vi "ODE_quaternion.vi"() -> ()   [LabVIEW 2018]
uses:
  <vilib>/robotics/Kinematics/Quaternion.ctl
  <vilib>/Analysis/_algsub.llb/Vector Norm.vi
  <vilib>/Analysis/_algsub.llb/Real Vector Norm.vi
  <vilib>/Analysis/baseanly.llb/Outer Product.vi
  <vilib>/Analysis/baseanly.llb/Real Outer Product.vi
  <vilib>/robotics/Kinematics/Create Lie Group Matrix.vi
  <vilib>/imath/engines/lvmath2/RunTimeEngine/Managers/WorkSpace/UID Generator.vi
  <vilib>/imath/engines/lvmath2/RunTimeEngine/IndexRead/NIMS V(S).vi
  <instcachedir>/0/NIMS V(S)_0488751826AF41519A22953C041130DC.lvgen/NIMS V(S)_0488751826AF41519A22953C041130DC_002.vi
  <vilib>/imathl/engines/lvmath/Functions/Error Handling/Create Error.vi
  <vilib>/imath/engines/lvmath2/RunTimeEngine/RunTimeType/NIMS_RunTimeType_From StrictType (excl LVString).vi
  <instcachedir>/0/NIMS_RunTimeType_From StrictType (excl LVString)_E7E34A65C99947108168652BAD14964D.lvgen/NIMS_RunTimeType_From StrictType (excl LVString)_E7E34A65C99947108168652BAD14964D_000.vi
  <vilib>/imath/engines/lvmath2/RunTimeEngine/LocalVariableDefStatement/MC_LocalVariableDefStatement_Display.vi
  <vilib>/imath/engines/lvmath2/RunTimeEngine/ArithmeticOperatorToken/NIMS_ArithmeticOperator_multmx(M,CV)-internal.vi
  <instcachedir>/0/NIMS_ArithmeticOperator_multmx(M,CV)-internal_5287250D8D1D4A3E9F77F5DF08D432E0.lvgen/NIMS_ArithmeticOperator_multmx(M,CV)-internal_5287250D8D1D4A3E9F77F5DF08D432E0_003.vi
  <instcachedir>/0/NIMS V(S)_0488751826AF41519A22953C041130DC.lvgen/NIMS V(S)_0488751826AF41519A22953C041130DC_000.vi
  <vilib>/imath/engines/lvmath2/RunTimeEngine/Managers/SymbolTable/Clear UID.vi
  <vilib>/imath/engines/lvmath2/RunTimeEngine/NodeEndStatement/NIMS_NodeEndStatement_Output.vi
  <instcachedir>/0/NIMS_NodeEndStatement_Output_53EC0D466D134D7ABD903AC30B43404B.lvgen/NIMS_NodeEndStatement_Output_53EC0D466D134D7ABD903AC30B43404B_005.vi
  <vilib>/imath/engines/lvmath2/RunTimeEngine/ErrorHandling/NIMS_Finalize Error.vi
  <vilib>/Analysis/Matrix/Numeric/Multiply/Multiply.vi
  <vilib>/Analysis/Matrix/Numeric/Multiply/Multiply - RM,R.vi
  <vilib>/Analysis/Matrix/Numeric/Multiply/Multiply - R,RM.vi
  <vilib>/Analysis/Matrix/Numeric/Add/Add.vi
  <vilib>/Analysis/Matrix/Numeric/Add/Add - RM,RM.vi
  <vilib>/Analysis/Matrix/Numeric/Conversions/Matrix To Array - RM.vi
  <vilib>/imath/engines/lvmath2/RunTimeEngine/IndexRead/NIMS M(S,S).vi
  <instcachedir>/0/NIMS M(S,S)_AC51E74150A542F7991B9634C66F3096.lvgen/NIMS M(S,S)_AC51E74150A542F7991B9634C66F3096_000.vi
  <vilib>/imath/engines/lvmath2/RunTimeEngine/BuiltInFunctions/abs/NIMS_abs(signed).vi
  <instcachedir>/0/NIMS_abs(signed)_C4FCB8E6058B49B797C7C8D53CA5F6EC.lvgen/NIMS_abs(signed)_C4FCB8E6058B49B797C7C8D53CA5F6EC_000.vi
  <vilib>/imath/engines/lvmath2/RunTimeEngine/BuiltInFunctions/atan2/NIMS_atan2.vi
  <instcachedir>/0/NIMS_atan2_A91AA4A7D42247EDBE8F76DB99AF04A4.lvgen/NIMS_atan2_A91AA4A7D42247EDBE8F76DB99AF04A4_002.vi
  <vilib>/imath/engines/lvmath2/RunTimeEngine/ErrorHandling/NIMS_Create Error From Enums.vi
  <vilib>/imath/engines/lvmath2/RunTimeEngine/BuiltInFunctions/cos/NIMS_cos(C).vi
  <instcachedir>/0/NIMS_cos(C)_96B8A70E6B8E4D29AD8526A89C8CF3DF.lvgen/NIMS_cos(C)_96B8A70E6B8E4D29AD8526A89C8CF3DF_001.vi
  <instcachedir>/0/NIMS_atan2_A91AA4A7D42247EDBE8F76DB99AF04A4.lvgen/NIMS_atan2_A91AA4A7D42247EDBE8F76DB99AF04A4_001.vi
  <vilib>/gmath/NI_Gmath.lvlib
  <vilib>/robotics/Kinematics/NI_Kinematics.lvlib
  <vilib>/imath/engines/lvmath2/RunTimeEngine/Managers/SymbolTable/NIMS_WorkSpace.lvlib
  <vilib>/Analysis/Matrix/NI_Matrix.lvlib
panel:
  out "E":dbl[](array[numeric])
  out "unit quaternion":T1
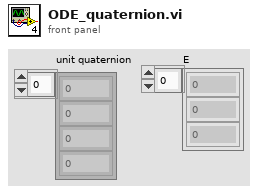
[diagram p1: front panel]
types:
  T1 = typedef "NI_Kinematics.lvlib/Quaternion.ctl" = dbl[]
  T2 = typedef "NI_Matrix.lvlib/RealMatrix.ctl" = dbl[][]
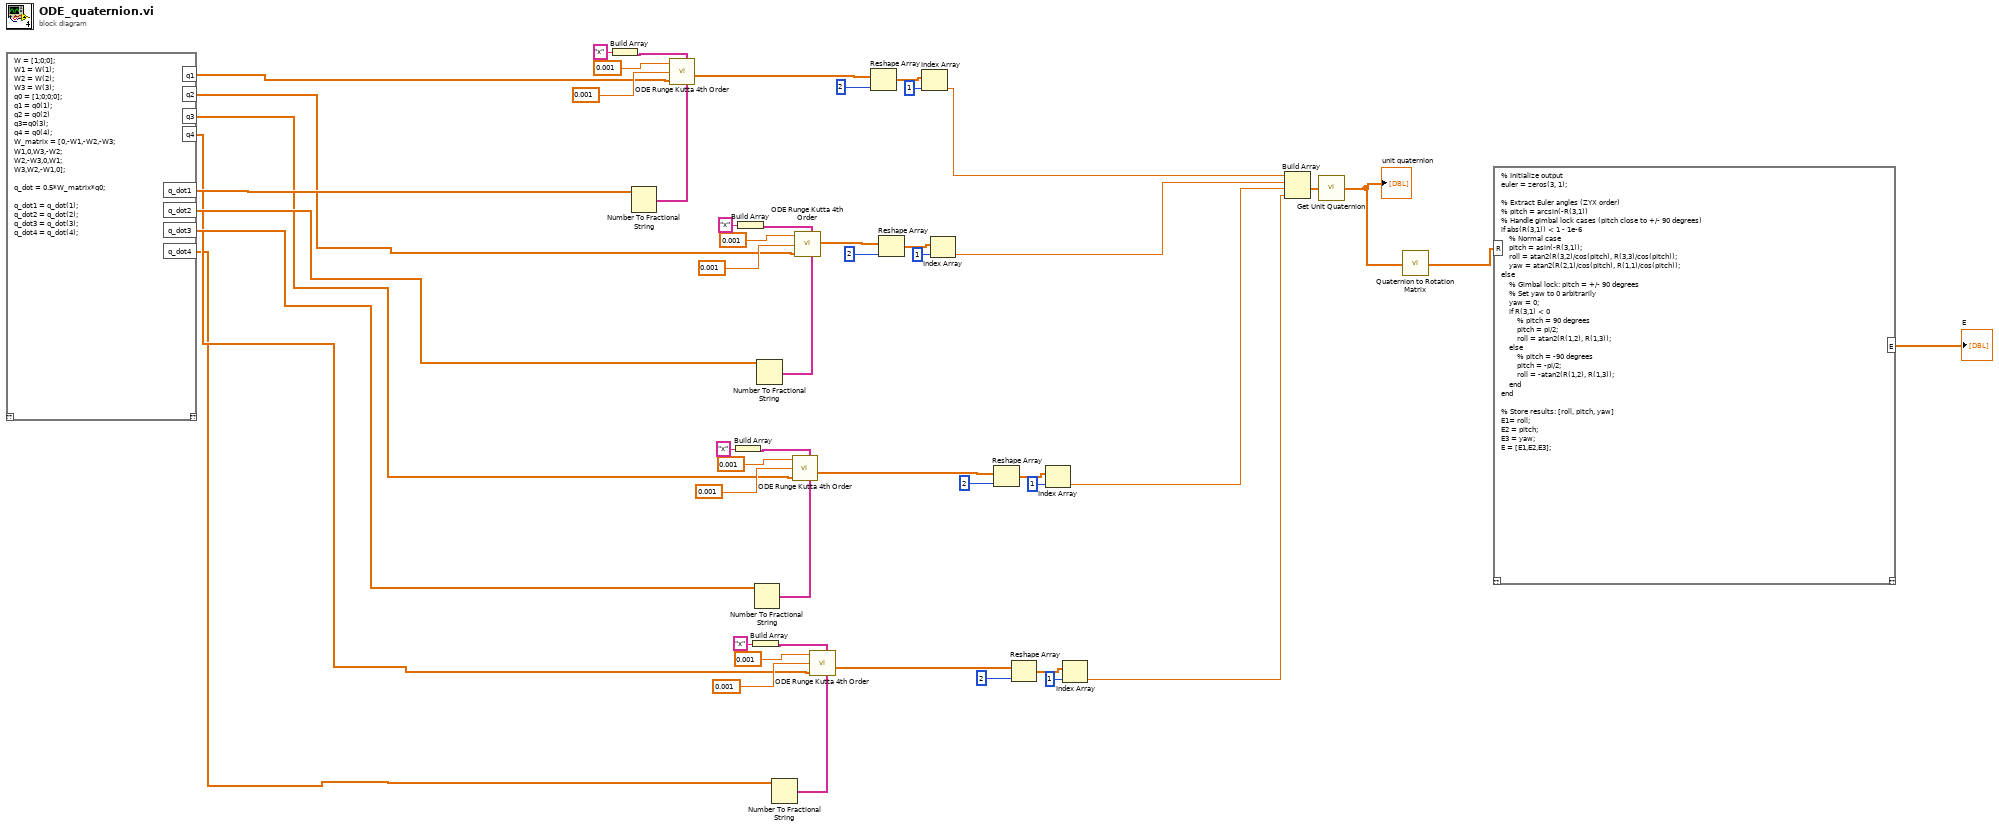
[diagram p0: block diagram]
diagram:
  n1 = mathscript code="W = [1;0;0];\nW1 = W(1);\nW2 = W(2);\nW3 = W(3);\nq0 = [1;0;0;0];\nq1 = q0(1);\nq2 = q0(2)\nq3=q0(3);\nq4 = q0(4);\nW_matrix = [0,-W1,-W2,-W3;\nW1,0,W3,-W2;\nW2,-W3,0,W1;\nW3,W2,-W1,0];\n\nq_dot = 0.5*W_matrix*q0;\n\nq_dot1 = q_dot(1);\nq_dot2 = q_dot(2);\nq_dot3 = q_dot(3);\nq_dot4 = q_dot(4);"() -> ("q_dot1"=w42:dbl[], "q_dot2"=w31:dbl[], "q_dot3"=w20:dbl[], "q_dot4"=w9:dbl[], "q1"=w43:dbl[], "q2"=w32:dbl[], "q3"=w21:dbl[], "q4"=w10:dbl[])  [unwired: 1 in, 1 out]
  n2 = Build Array("x") -> (w51:string[])
  n3 = Number To Fractional String(number=w42) -> (F-format string=w48:string[])  [unwired: 3 in]
  n4 = call <vilib>:"ODE Runge Kutta 4th Order.vi"("time end"=0.001, "h (step rate)"=0.001, "X0"=w43, "X (name of variables)"=w51, "F(X,t) (right sides of the ODE\nas functions of X and t)"=w48) -> ("X Values (solution)"=w44:dbl[][])  [unwired: 2 in, 3 out]
  n5 = Build Array("x") -> (w29:string[])
  n6 = Build Array("x") -> (w40:string[])
  n7 = Build Array("x") -> (w18:string[])
  n8 = Number To Fractional String(number=w20) -> (F-format string=w26:string[])  [unwired: 3 in]
  n9 = Number To Fractional String(number=w31) -> (F-format string=w37:string[])  [unwired: 3 in]
  n10 = Number To Fractional String(number=w9) -> (F-format string=w15:string[])  [unwired: 3 in]
  n11 = call <vilib>:"ODE Runge Kutta 4th Order.vi"("time end"=0.001, "h (step rate)"=0.001, "X0"=w21, "X (name of variables)"=w29, "F(X,t) (right sides of the ODE\nas functions of X and t)"=w26) -> ("X Values (solution)"=w22:dbl[][])  [unwired: 2 in, 3 out]
  n12 = call <vilib>:"ODE Runge Kutta 4th Order.vi"("time end"=0.001, "h (step rate)"=0.001, "X0"=w32, "X (name of variables)"=w40, "F(X,t) (right sides of the ODE\nas functions of X and t)"=w37) -> ("X Values (solution)"=w33:dbl[][])  [unwired: 2 in, 3 out]
  n13 = call <vilib>:"ODE Runge Kutta 4th Order.vi"("time end"=0.001, "h (step rate)"=0.001, "X0"=w10, "X (name of variables)"=w18, "F(X,t) (right sides of the ODE\nas functions of X and t)"=w15) -> ("X Values (solution)"=w11:dbl[][])  [unwired: 2 in, 3 out]
  n14 = Reshape Array(w44, 2 ("dimension size")) -> (w46:dbl[])
  n15 = Reshape Array(w33, 2 ("dimension size")) -> (w35:dbl[])
  n16 = Index Array(array=w46, index=1) -> (element=w8:dbl)
  n17 = Index Array(array=w35, index=1) -> (element=w7:dbl)
  n18 = Reshape Array(w22, 2 ("dimension size")) -> (w24:dbl[])
  n19 = Reshape Array(w11, 2 ("dimension size")) -> (w13:dbl[])
  n20 = Index Array(array=w24, index=1) -> (element=w6:dbl)
  n21 = Index Array(array=w13, index=1) -> (element=w5:dbl)
  n22 = Build Array(w8, w7, w6, w5) -> (w4:dbl[])
  n23 = call <vilib>:"Get Unit Quaternion.vi"("quaternion"=w4) -> ("unit quaternion"=w3:T1)
  "unit quaternion" <- w3
  n24 = call <vilib>:"Quaternion to Rotation Matrix.vi"("quaternion"=w3) -> ("rotation matrix"=w2:T2)
  n25 = mathscript code="% Initialize output\neuler = zeros(3, 1);\n\n% Extract Euler angles (ZYX order)\n% pitch = arcsin(-R(3,1))\n% Handle gimbal lock cases (pitch close to +/- 90 degrees)\nif abs(R(3,1)) < 1 - 1e-6\n    % Normal case\n    pitch = asin(-R(3,1));\n    roll = atan2(R(3,2)/cos(pitch), R(3,3)/cos(pitch));\n    yaw = atan2(R(2,1)/cos(pitch), R(1,1)/cos(pitch));\nelse\n    % Gimbal lock: pitch = +/- 90 degrees\n    % Set yaw to 0 arbitrarily\n    yaw = 0;\n    if R(3,1) < 0\n        % pitch = 90 degrees\n        pitch = pi/2;\n        roll = atan2(R(1,2), R(1,3));\n    else\n        % pitch = -90 degrees\n        pitch = -pi/2;\n        roll = -atan2(R(1,2), R(1,3));\n    end\nend\n\n% Store results: [roll, pitch, yaw]\nE1= roll;\nE2 = pitch;\nE3 = yaw;\nE = [E1,E2,E3];"("R"=w2) -> ("E"=→"E":dbl[])  [unwired: 1 in, 1 out]
